vi "CheckAndOpenFpga.vi"(8 "error in (no error)":errorcluster, 11 "SETI_LV_FPGA in":refnum<class "SETI_LV_FPGA.lvclass">) -> (0 "error out":errorcluster, 3 "SETI_LV_FPGA out":refnum<class "SETI_LV_FPGA.lvclass">)   [LabVIEW 2015, in "SETI_LV_FPGA.lvclass"]
uses:
  SETI_LV_FPGA.lvclass
  SETI_LV_FPGA.lvclass/SETI_LV_FPGA.ctl
  <vilib>/rvi/interface/RandomDataEmulation/nirviRandomDataOpen.vi
  <vilib>/rvi/errors/niLvFpgaMergeErrorWithErrorCode.vi
  <vilib>/rvi/interface/RandomDataEmulation/nirviRandomDataRunMethod.vi
  <vilib>/rvi/interface/RandomDataEmulation/nirviRandomDataDMAMethods.vi
  <vilib>/rvi/interface/nirviOpenFPGA/nirviOpenFPGA.xnode
  Fpga-Version/PXI-7953R/Fft.vi
  <vilib>/rvi/interface/nirviMethod/nirviMethod.xnode
  <vilib>/FPGA/interface/niFpgaViExecutionMode.ctl
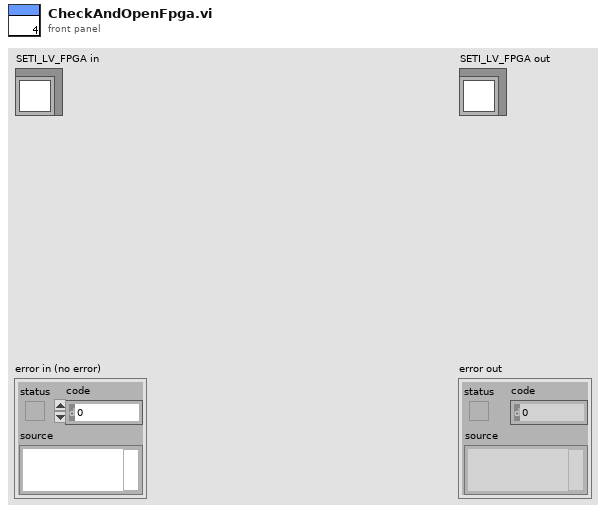
[diagram p1: front panel]
types:
  T1 = typedef "niFpgaViExecutionMode.ctl" = enum16{"FPGA Target", "Simulation (Simulated I/O)", "Simulation (Real I/O)", "Third-Party Simulation"}
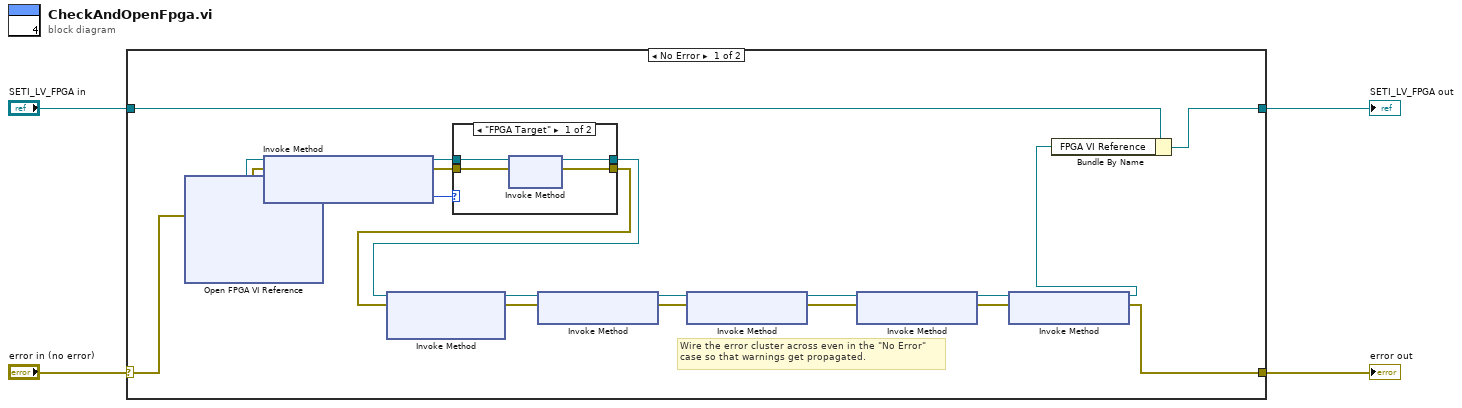
[diagram p0: block diagram]
diagram:
  n1 = case shown="No Error" "error in (no error)" {
    selector: "error in (no error)" -> [w9 w32]
    tunnel: [w8 w32] -> w3
    tunnel: [w6 w31] -> w1
    tunnel: "SETI_LV_FPGA in" -> [w7 w31]
    frame No Error {
      # "Wire the error cluster across even in the \"No Error\"\ncase so that warnings get propagated."
      n2 = xnode "Open FPGA VI Reference"("error in"=w9) -> ("FPGA VI Reference Out"=w22:refnum<k20>, "error out"=w17:errorcluster)  [unwired: 1 in]
      n3 = xnode "Invoke Method"("FPGA VI Reference In"=w22, "error in"=w17) -> ("FPGA VI Reference Out"=w20:refnum<k20>, "error out"=w19:errorcluster, "FPGA VI Execution Mode"=w21:T1)
      n4 = case shown="\"FPGA Target\"" w21 {
        tunnel: [w28 w29] -> w15
        tunnel: [w27 w30] -> w18
        tunnel: w20 -> [w26 w30]
        tunnel: w19 -> [w25 w29]
        frame "FPGA Target" {
          n5 = xnode "Invoke Method"("FPGA VI Reference In"=w26, "error in"=w25) -> ("FPGA VI Reference Out"=w27:refnum<k20>, "error out"=w28:errorcluster)
        }
        frame "Simulation (Simulated I/O)", Default {
        }
      }
      n6 = xnode "Invoke Method"("FPGA VI Reference In"=w18, "error in"=w15) -> ("FPGA VI Reference Out"=w16:refnum<k20>, "error out"=w10:errorcluster)  [unwired: 1 in]
      n7 = xnode "Invoke Method"("FPGA VI Reference In"=w16, "error in"=w10) -> ("FPGA VI Reference Out"=w14:refnum<k20>, "error out"=w11:errorcluster)
      n8 = xnode "Invoke Method"("FPGA VI Reference In"=w14, "error in"=w11) -> ("FPGA VI Reference Out"=w13:refnum<k20>, "error out"=w12:errorcluster)
      n9 = xnode "Invoke Method"("FPGA VI Reference In"=w13, "error in"=w12) -> ("FPGA VI Reference Out"=w23:refnum<k20>, "error out"=w24:errorcluster)
      n10 = xnode "Invoke Method"("FPGA VI Reference In"=w23, "error in"=w24) -> ("FPGA VI Reference Out"=w5:refnum<k20>, "error out"=w8:errorcluster)
      n11 = Bundle By Name(cluster=w7, "FPGA VI Reference"=w5) -> (w6:refnum<class "SETI_LV_FPGA.lvclass">)
    }
    frame Error {
    }
  }
  "error out" <- w3
  "SETI_LV_FPGA out" <- w1
